vi "GateRefSelector.vi"(10 "GateRefs":T1) -> (2 "Refnum":string)   [LabVIEW 2014, in "GateLib.lvlib"]
uses:
  GateLib.lvlib
  GateRefs.ctl
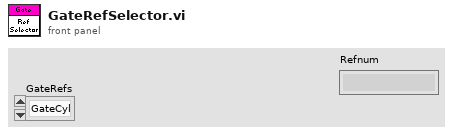
[diagram p1: front panel]
types:
  T1 = typedef "GateLib.lvlib/GateRefs.ctl" = enum16{"GateCyl"}
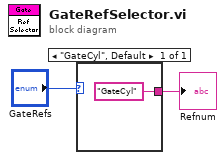
[diagram p0: block diagram]
diagram:
  n1 = case shown="\"GateCyl\", Default" "GateRefs" {
    tunnel: ["GateCyl"] -> w1
    frame "GateCyl", Default {
    }
  }
  "Refnum" <- w1
